vi "ReadWaveform(subVI).vi"(2 "Handle":i32, 3 "ADC Rate (ms)":dbl=1.0 min=0.033333 max=5.0 format="%.4f", 4 "Number of position values":u32=2 min=2 max=1000, 5 "Axis":u32) -> (0 "Data Array":dbl[](array[numeric]) format="%.4f", 1 "Return Code":i32)   [LabVIEW 2012]
uses:
  Madlib.dll
panel:
  out "String":string
  # "This example demonstrates reading a series (array) of positions in a single step."
  # "X = 1\nY = 2\nZ = 3"
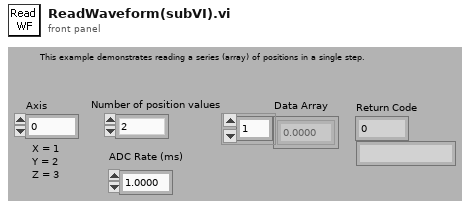
[diagram p1: front panel]
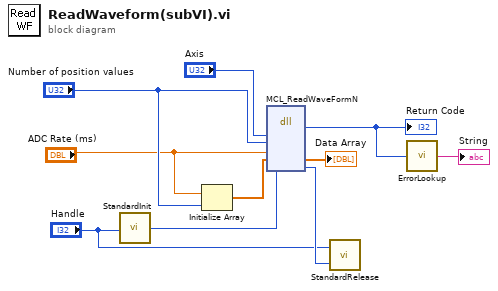
[diagram p0: block diagram]
diagram:
  n1 = call "StandardInit.vi"("Incoming Handle"="Handle") -> ("Outgoing Handle"=w6:i32)
  n2 = Initialize Array "Initialize Array"("ADC Rate (ms)", "Number of position values") -> (w10:dbl[])
  n3 = dll-call lib="C:/Users/Labview/Desktop/SRR/Madlib_x64/Labview Examples/MADLib.dll" fn="MCL_ReadWaveFormN"("axis"="Axis", "DataPoints"="Number of position values", "milliseconds"="ADC Rate (ms)", "waveform"=w10, "handle"=w6) -> (w2:i32, "waveform"=→"Data Array":dbl[], "handle"=w4:i32)  [unwired: 6 in, 2 out]
  "Return Code" <- w2
  n4 = call "StandardRelease.vi"("Outgoing Handle"=w4, "Incoming Handle"="Handle") -> ()  [unwired: 1 in]
  n5 = call "ErrorLookup.vi"("Error Code"=w2) -> ("Error"=→"String":string)
